vi "Read TaskConfig.vi"(8 "error in (no error)":errorcluster, 11 "Task_Abstr in":refnum<class "Task_Abstr.lvclass">) -> (0 "error out":errorcluster, 2 "TaskConfig":T1={"TaskType"=enum."AI", "PhysicalChannels"="", "SampleRateConfiguration"={"SampleRate"=0.0, "SamplesPerChannel"=0, "SamplesPerRead"=0, "SampleMode"=10123, "Clock Source"="OnboardClock"}, "ChannelConfig"=""} {"SampleRateConfiguration"."SampleMode" items=["Finite Samples"=10178, "Continuous Samples"=10123, "Hardware Timed Single Point"=12522]}, 3 "Task_Abstr out":refnum<class "Task_Abstr.lvclass">)   [LabVIEW 2025, in "Task_Abstr.lvlib" / "Task_Abstr.lvclass"]
uses:
  Task_Abstr.lvclass
  DAQ_Module/DAQ_Module/DAQ_Module/DAQ_Task_Config.ctl
  DAQ_Module/DAQ_Module/DAQ_Module/DAQ_Task_Type.ctl
  Task_Abstr.lvclass/Task_Abstr.ctl
  DAQ_Module/DAQ_Module/DAQ_Module/DAQ_Module.lvclass
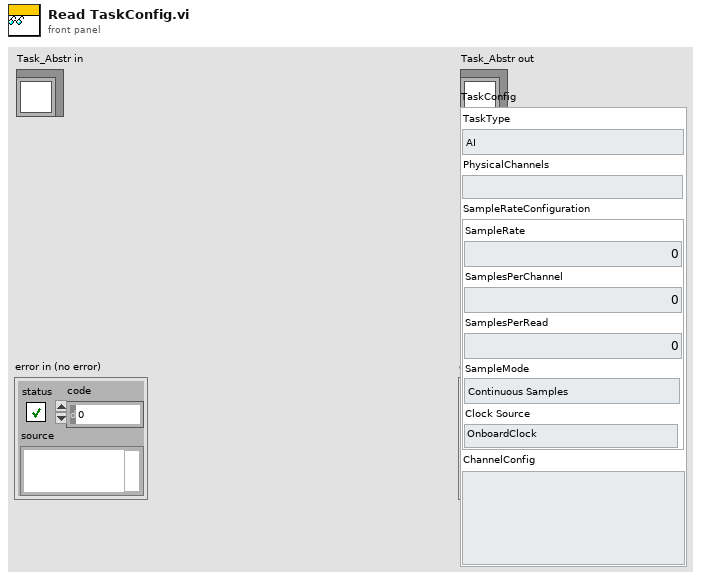
[diagram p1: front panel]
types:
  T1 = typedef "DAQ_Module.lvlib/DAQ_Module.lvclass/DAQ_Task_Config.ctl" = cluster{"TaskType":T2, "PhysicalChannels":string, "SampleRateConfiguration":cluster{"SampleRate":dbl, "SamplesPerChannel":u32, "SamplesPerRead":i32, "SampleMode":i32, "Clock Source":string}, "ChannelConfig":string}
  T2 = typedef "DAQ_Module.lvlib/DAQ_Module.lvclass/DAQ_Task_Type.ctl" = enum16{"AI", "Linear", "Angular", "AO"}
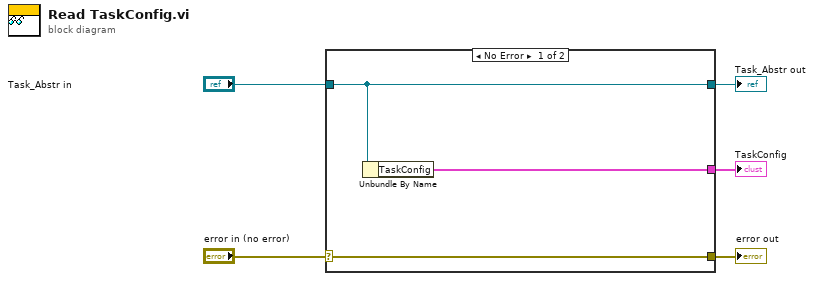
[diagram p0: block diagram]
diagram:
  n1 = case shown="No Error" "error in (no error)" {
    selector: "error in (no error)" -> [w8 w9]
    tunnel: [w8 w9] -> w4
    tunnel: [w7 w10] -> w2
    tunnel: "Task_Abstr in" -> [w7 w10]
    tunnel: [w6 _] -> w1
    frame No Error {
      n2 = Unbundle By Name(w7) -> ("TaskConfig"=w6:T1)
    }
    frame Error {
    }
  }
  "error out" <- w4
  "Task_Abstr out" <- w2
  "TaskConfig" <- w1
